vi "HEWH_DSM_CMD.vi"(10 "Command":T1=34 items=["RQST_SOFTWARE_VERSION", "RQST_T2_RESISTANCE", "RQST_T3A_RESISTANCE", "RQST_T3B_RESISTANCE", "RQST_T4_RESISTANCE", "RQST_T5_RESISTANCE", "RQST_IDLB_RESISTANCE", "RQST_MODE_SELECT_RESISTANCE", "RQST_DATA_FROM_MEMORY", "RQST_DATA_FROM_DATA_FLASH", "RQST_SS_FAULT_COUNTS", "RQST_OTHER_FAULT_COUNTS", "CMD_CLEAR_FAULT_COUNTS", "RQST_HYPERTERM_OUTPUT_DATA", "CMD_RESET_FILTER_TIMES", "CMD_WRITE_SETPOINTS", "CMD_TURN_ON_OFF_DLB", "CMD_ENTER_EXIT_FCT_MODE", "CMD_SET_LEDS", "CMD_SET_EEV_DRIVE_LINES", "REQ_READ_KEY_STATUS", "RQST_READ_PERSONALITY", "CMD_ENTER_FACT_MODE", "CMD_RESET", "CMD_RESTORE_EEPROM_DEFAULTS", "CMD_SET_MODEL_NUMBER", "CMD_SET_SERIAL_NUMBER", "RQST_MODEL_NUMBER", "RQST_SERIAL_NUMBER", "CMD_TOGGLE_SERVICE_MODE", "CMD_TOGGLE_UE_SERV", "CMD_TOGGLE_LE_SERV", "CMD_REFRESH_SERVICE_TIMEOUTS", "RQST_DSM_OVERRIDE_STATUS", "RQST_STATUS_QUERY", "RQST_HEM_KWH_DATA", "RQST_SERVICE_ERROR_CODES", "RQST_OVERRIDE_STATUS", "CMD_UPDATE_DSM_LEVEL", "CMD_OVERRIDE_STATUS_CHANGED", "CMD_CLEAR_OVERRIDE_STATUS", "CMD_CLEAR_ENERGY_USAGE_CTRS", "CMD_DSM_OVERRIDES", "CMD_UPDATE_MODE", "CMD_SET_PID_P_DENOMINATOR", "CMD_SET_PID_I_DENOM_UNDER_THR", "CMD_SET_PID_I_DENOM_OVER_THR", "CMD_SET_START_POS_UNDER_THR", "CMD_SET_START_POS_OVER_THR", "CMD_SET_EEV_STOP_POSITION", "CMD_SET_AMBIENT_THRESH_1", "CMD_SET_AMBIENT_THRESH_2", "CMD_SET_AMBIENT_THRESH_3", "CMD_SET_PID_LOW_SH_TARGET", "CMD_SET_PID_MID_SH_TARGET", "RQST_PID_PARAMETERS", "CMD_COMP_OFF", "CMD_TOGGLE_FAN", "CMD_RQST_LED_STATUS", "CMD_UE_2_SECONDS", "CMD_LE_2_SECONDS", "CMD_COMP_ON", "CMD_HP_RUN_6MIN", "RQST_TEMP_RANGE", "RQST_VACATION_RANGE", "RQST_STD_ELEC_RANGE", "RQST_WATER_CAPACITY", "CMD_CANCEL_EEV_POSITION", "CMD_EEV_POSITION", "CMD_SET_CURRENTS", "RQST_SUPPORTED_MODES"]) -> (2 "CMD Array":u8[](array[numeric])=[222, 2] format="%02x")   [LabVIEW 2009]
uses:
  HEWH Command Type.ctl
panel:
  in  "Commands":cluster{"String":string, "CMD Array":u8[]}[](array[cluster])=[{"String"="RQST_SOFTWARE_VERSION", "CMD Array"=[1]}, {"String"="RQST_T2_RESISTANCE", "CMD Array"=[16]}, {"String"="RQST_T3A_RESISTANCE", "CMD Array"=[17]}, {"String"="RQST_T3B_RESISTANCE", "CMD Array"=[18]}, {"String"="RQST_T4_RESISTANCE", "CMD Array"=[19]}, {"String"="RQST_T5_RESISTANCE", "CMD Array"=[20]}, {"String"="RQST_IDLB_RESISTANCE", "CMD Array"=[21]}, {"String"="RQST_MODE_SELECT_RESISTANCE", "CMD Array"=[22]}, {"String"="RQST_DATA_FROM_MEMORY", "CMD Array"=[78]}, {"String"="RQST_DATA_FROM_DATA_FLASH", "CMD Array"=[79]}, {"String"="RQST_SS_FAULT_COUNTS", "CMD Array"=[83]}, {"String"="RQST_OTHER_FAULT_COUNTS", "CMD Array"=[84]}, {"String"="CMD_CLEAR_FAULT_COUNTS", "CMD Array"=[85]}, {"String"="RQST_HYPERTERM_OUTPUT_DATA", "CMD Array"=[86]}, {"String"="CMD_RESET_FILTER_TIMES", "CMD Array"=[144]}, {"String"="CMD_WRITE_SETPOINTS", "CMD Array"=[165]}, {"String"="CMD_TURN_ON_OFF_DLB", "CMD Array"=[176]}, {"String"="CMD_ENTER_EXIT_FCT_MODE", "CMD Array"=[180]}, {"String"="CMD_SET_LEDS", "CMD Array"=[181]}, {"String"="CMD_SET_EEV_DRIVE_LINES", "CMD Array"=[182]}, {"String"="REQ_READ_KEY_STATUS", "CMD Array"=[183]}, {"String"="RQST_READ_PERSONALITY", "CMD Array"=[188]}, {"String"="CMD_ENTER_FACT_MODE", "CMD Array"=[192]}, {"String"="CMD_RESET", "CMD Array"=[193]}, {"String"="CMD_RESTORE_EEPROM_DEFAULTS", "CMD Array"=[194]}, {"String"="CMD_SET_MODEL_NUMBER", "CMD Array"=[195]}, {"String"="CMD_SET_SERIAL_NUMBER", "CMD Array"=[196]}, {"String"="RQST_MODEL_NUMBER", "CMD Array"=[197]}, {"String"="RQST_SERIAL_NUMBER", "CMD Array"=[198]}, {"String"="CMD_TOGGLE_SERVICE_MODE", "CMD Array"=[200]}, {"String"="CMD_TOGGLE_UE_SERV", "CMD Array"=[201]}, {"String"="CMD_TOGGLE_LE_SERV", "CMD Array"=[202]}, {"String"="CMD_REFRESH_SERVICE_TIMEOUTS", "CMD Array"=[203]}, {"String"="RQST_DSM_OVERRIDE_STATUS", "CMD Array"=[222, 2]}, {"String"="RQST_STATUS_QUERY", "CMD Array"=[222, 16]}, {"String"="RQST_HEM_KWH_DATA", "CMD Array"=[222, 18]}, {"String"="RQST_SERVICE_ERROR_CODES", "CMD Array"=[222, 20]}, {"String"="RQST_OVERRIDE_STATUS", "CMD Array"=[222, 23]}, {"String"="CMD_UPDATE_DSM_LEVEL", "CMD Array"=[223, 0]}, {"String"="CMD_OVERRIDE_STATUS_CHANGED", "CMD Array"=[223, 2]}, {"String"="CMD_CLEAR_OVERRIDE_STATUS", "CMD Array"=[223, 3]}, {"String"="CMD_CLEAR_ENERGY_USAGE_CTRS", "CMD Array"=[223, 7]}, {"String"="CMD_DSM_OVERRIDES", "CMD Array"=[223, 19]}, {"String"="CMD_UPDATE_MODE", "CMD Array"=[223, 20]}, {"String"="CMD_SET_PID_P_DENOMINATOR", "CMD Array"=[0]}, {"String"="CMD_SET_PID_I_DENOM_UNDER_THR", "CMD Array"=[0]}, {"String"="CMD_SET_PID_I_DENOM_OVER_THR", "CMD Array"=[0]}, {"String"="CMD_SET_START_POS_UNDER_THR", "CMD Array"=[0]}, {"String"="CMD_SET_START_POS_OVER_THR", "CMD Array"=[0]}, {"String"="CMD_SET_EEV_STOP_POSITION", "CMD Array"=[0]}, {"String"="CMD_SET_AMBIENT_THRESH_1", "CMD Array"=[0]}, {"String"="CMD_SET_AMBIENT_THRESH_2", "CMD Array"=[0]}, {"String"="CMD_SET_AMBIENT_THRESH_3", "CMD Array"=[0]}, {"String"="CMD_SET_PID_LOW_SH_TARGET", "CMD Array"=[0]}, {"String"="CMD_SET_PID_MID_SH_TARGET", "CMD Array"=[0]}, {"String"="RQST_PID_PARAMETERS", "CMD Array"=[0]}, {"String"="CMD_COMP_OFF", "CMD Array"=[240]}, {"String"="CMD_TOGGLE_FAN", "CMD Array"=[241]}, {"String"="CMD_RQST_LED_STATUS", "CMD Array"=[242]}, {"String"="CMD_UE_2_SECONDS", "CMD Array"=[243]}, {"String"="CMD_LE_2_SECONDS", "CMD Array"=[244]}, {"String"="CMD_COMP_ON", "CMD Array"=[245]}, {"String"="CMD_HP_RUN_6MIN", "CMD Array"=[246]}, {"String"="RQST_TEMP_RANGE", "CMD Array"=[247]}, {"String"="RQST_VACATION_RANGE", "CMD Array"=[248]}, {"String"="RQST_STD_ELEC_RANGE", "CMD Array"=[249]}, {"String"="RQST_WATER_CAPACITY", "CMD Array"=[250]}, {"String"="CMD_CANCEL_EEV_POSITION", "CMD Array"=[251]}, {"String"="CMD_EEV_POSITION", "CMD Array"=[252]}, {"String"="CMD_SET_CURRENTS", "CMD Array"=[253]}, {"String"="RQST_SUPPORTED_MODES", "CMD Array"=[254]}] {"CMD Array" format="%.0x"}
  out "Data Array":string[][](array[string])=[["CMD_WRITE_SETPOINTS", "0x60", "0xA5", "N/A", "Any"], ["RQST_NON_CRIT_VERSION", "0x60", "0x01", "N/A", "Any"], ["RQST_CRIT_VERSION", "0x60", "0x02", "N/A", "Any"], ["RQST_EEPROM_VERSION", "0x60", "0x03", "N/A", "Any"], ["RQST_T2_RESISTANCE", "0x60", "0x10", "N/A", "Any"], ["RQST_T3A_RESISTANCE", "0x60", "0x11", "N/A", "Any"], ["RQST_T3B_RESISTANCE", "0x60", "0x12", "N/A", "Any"], ["RQST_T4_RESISTANCE", "0x60", "0x13", "N/A", "Any"], ["RQST_T5_RESISTANCE", "0x60", "0x14", "N/A", "Any"], ["RQST_IDLB_RESISTANCE", "0x60", "0x15", "N/A", "Any"], ["RQST_MODE_SELECT_RESISTANCE", "0x60", "0x16", "N/A", "Any"], ["RQST_STATUS INFO", "0x60", "0x50", "N/A", "Any"], ["RQST_SS_FAULT_COUNTS", "0x60", "0x53", "N/A", "Any"], ["RQST_OTHER_FAULT_COUNTS", "0x60", "0x54", "N/A", "Any"], ["CMD_CLEAR_FAULT_COUNTS", "0x60", "0x55", "N/A", "Any"], ["RQST_HYPERTERM_OUTPUT_DATA", "0x60", "0x56", "N/A", "Any"], ["RQST_READ_PERSONALITY", "0x60", "0xBC", "N/A", "Any"], ["RQST_DSM_OVERRIDE_STATUS", "0x60", "0xDE", "0x02", "Any"], ["RQST_STATUS_QUERY", "0x60", "0xDE", "0x10", "Any"], ["RQST_HEM_KWH_DATA", "0x60", "0xDE", "0x12", "Any"], ["RQST_SERVICE_ERROR_CODES", "0x60", "0xDE", "0x14", "Any"], ["RQST_OVERRIDE_STATUS", "0x60", "0xDE", "0x17", "Any"], ["CMD_CLEAR_OVERRIDE_STATUS", "0x60", "0xDF", "0x03", "0x40"], ["CMD_CLEAR_ENERGY_USAGE_CTRS", "0x60", "0xDF", "0x07", "0x40"], ["CMD_COMP_OFF", "0x60", "0xF0", "N/A", "Any"], ["CMD_UE_2_SECONDS", "0x60", "0xF3", "N/A", "Any"], ["CMD_LE_2_SECONDS", "0x60", "0xF4", "N/A", "Any"], ["CMD_COMP_ON", "0x60", "0xF5", "N/A", "Any"], ["CMD_HP_RUN_6MIN", "0x60", "0xF6", "N/A", "Any"], ["RQST_TEMP_RANGE", "0x60", "0xF7", "N/A", "Any"], ["RQST_VACATION_RANGE", "0x60", "0xF8", "N/A", "Any"], ["RQST_STD_ELEC_RANGE", "0x60", "0xF9", "N/A", "Any"], ["RQST_WATER_CAPACITY", "0x60", "0xFA", "N/A", "Any"], ["CMD_CANCEL_EEV_POSITION", "0x60", "0xFB", "N/A", "Any"], ["RQST_SUPPORTED_MODES", "0x60", "0xFE", "N/A", "Any"], ["CMD_CONTROL_FAN1", "0x60", "0xF1", "N/A", "Any"], ["CMD_EEV_POSITION", "0x60", "0xFC", "N/A", "Any"], ["CMD_SET_EEV_START_POSITION", "0x60", "E5", "N/A", "Any"], ["CMD_SET_EEV_STOP_POSITION", "0x60", "EA", "N/A", "Any"], ["CMD_UPDATE_DSM_LEVEL", "0x60", "0xDF", "0x00", "0x40"], ["CMD_SET_PID_I_DENOMINATOR", "0x60", "E3", "N/A", "Any"], ["CMD_SET_PID_I_NUMERATOR", "0x60", "E2", "N/A", "Any"], ["RQST_DATA_FROM_MEMORY", "0x60", "0x4E", "N/A", "Any"], ["CMD_OVERRIDE_STATUS_CHANGED", "0x40", "0xDF", "0x02", "0x60"], ["CMD_SET_PID_P_DENOMINATOR", "0x60", "E1", "N/A", "Any"], ["CMD_SET_PID_P_NUMERATOR", "0x60", "E0", "N/A", "Any"], ["CMD_SET_PID_RUN_SH_TARGET", "0x60", "E9", "N/A", "Any"], ["CMD_SET_PID_START_DWELL_TIME", "0x60", "E6", "N/A", "Any"], ["CMD_SET_PID_TRANSITION_TIME", "0x60", "E8", "N/A", "Any"], ["CMD_SET_PID_TRANS_SH_TARGET", "0x60", "E7", "N/A", "Any"], ["CMD_SET_PID_UPDATE_RATE", "0x60", "E4", "N/A", "Any"], ["RQST_DATA_FROM_DATA_FLASH", "0x60", "0x4F", "N/A", "Any"], ["CMD_DSM_OVERRIDES", "0x60", "0xDF", "0x13", "Any"], ["CMD_UPDATE_MODE", "0x60", "0xDF", "0x14", "Any"], ["CMD_UPDATE_SPECIAL_OPERATION", "0x60", "0xDF", "0x15", "Any"], ["CMD_SET_CURRENTS", "0x60", "0xFD", "N/A", "Any"], ["CMD_RESET_FILTER_TIMES", "0x60", "0x90", "N/A", "Any"], ["CMD_TURN_ON_DLB", "0x60", "B0", "N/A", "Any"], ["RQST_PID_PARAMETERS", "0x60", "EF", "N/A", "Any"], ["CMD_CHECK_CRC", "0x60", "0xA6", "N/A", "Any"], ["CMD_ENTER_FACT_MODE", "0x60", "0xC0", "N/A", "Any"], ["CMD_RESET", "0x60", "0xC1", "N/A", "Any"], ["CMD_RESTORE_EEPROM_DEFAULTS", "0x60", "0xC2", "N/A", "Any"]]
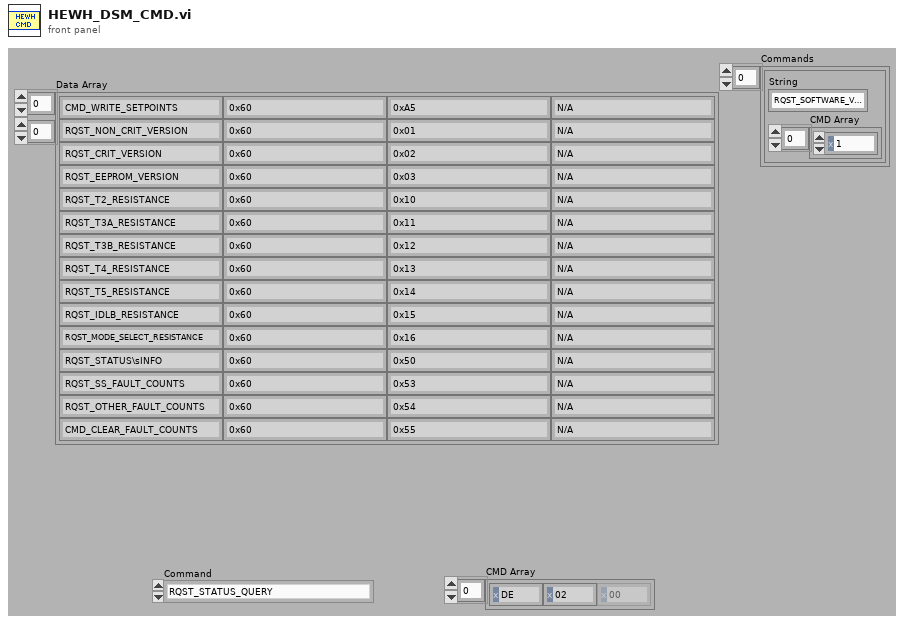
[diagram p1: front panel]
types:
  T1 = typedef "HEWH Command Type.ctl" = u8
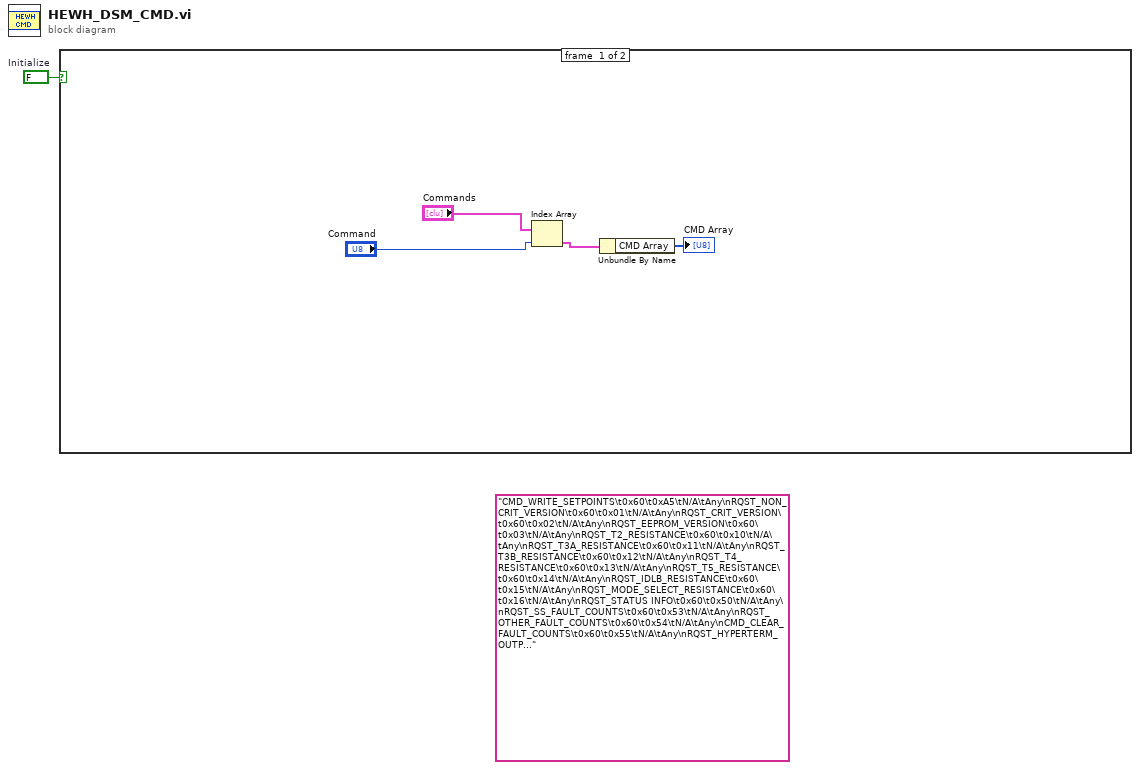
[diagram p0: block diagram]
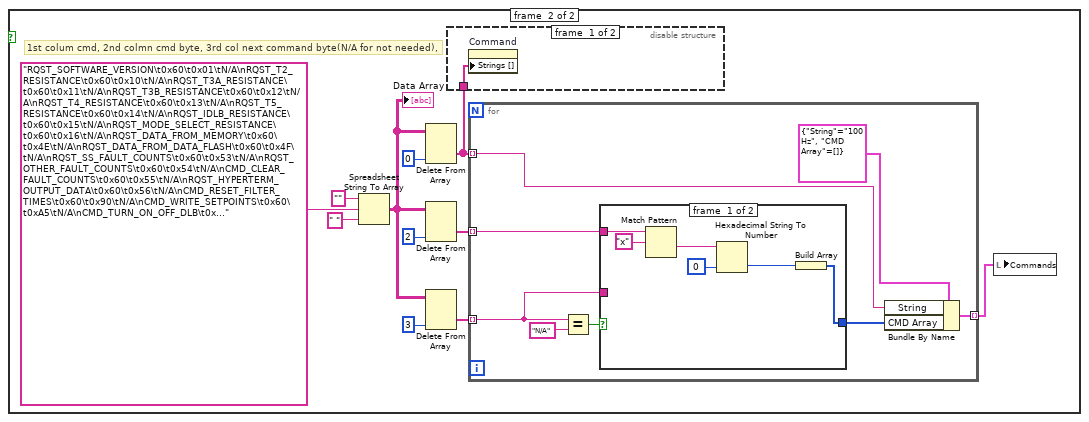
[diagram p2: hidden frame]
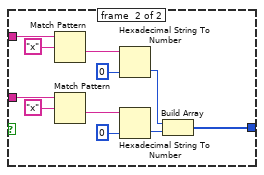
[diagram p4: hidden frame]
diagram:
  (unwired) "CMD_WRITE_SETPOINTS\t0x60\t0xA5\tN/A\tAny\nRQST_NON_CRIT_VERSION\t0x60\t0x01\tN/A\tAny\nRQST_CRIT_VERSION\t0x60\t0x02\tN/A\tAny\nRQST_EEPROM_VERSION\t0x60\t0x03\tN/A\tAny\nRQST_T2_RESISTANCE\t0x60\t0x10\tN/A\tAny\nRQST_T3A_RESISTANCE\t0x60\t0x11\tN/A\tAny\nRQST_T3B_RESISTANCE\t0x60\t0x12\tN/A\tAny\nRQST_T4_RESISTANCE\t0x60\t0x13\tN/A\tAny\nRQST_T5_RESISTANCE\t0x60\t0x14\tN/A\tAny\nRQST_IDLB_RESISTANCE\t0x60\t0x15\tN/A\tAny\nRQST_MODE_SELECT_RESISTANCE\t0x60\t0x16\tN/A\tAny\nRQST_STATUS INFO\t0x60\t0x50\tN/A\tAny\nRQST_SS_FAULT_COUNTS\t0x60\t0x53\tN/A\tAny\nRQST_OTHER_FAULT_COUNTS\t0x60\t0x54\tN/A\tAny\nCMD_CLEAR_FAULT_COUNTS\t0x60\t0x55\tN/A\tAny\nRQST_HYPERTERM_OUTPUT_DATA\t0x60\t0x56\tN/A\tAny\nRQST_READ_PERSONALITY\t0x60\t0xBC\tN/A\tAny\nRQST_DSM_OVERRIDE_STATUS\t0x60\t0xDE\t0x02\tAny\nRQST_STATUS_QUERY\t0x60\t0xDE\t0x10\tAny\nRQST_HEM_KWH_DATA\t0x60\t0xDE\t0x12\tAny\nRQST_SERVICE_ERROR_CODES\t0x60\t0xDE\t0x14\tAny\nRQST_OVERRIDE_STATUS\t0x60\t0xDE\t0x17\tAny\nCMD_CLEAR_OVERRIDE_STATUS\t0x60\t0xDF\t0x03\t0x40\nCMD_CLEAR_ENERGY_USAGE_CTRS\t0x60\t0xDF\t0x07\t0x40\nCMD_COMP_OFF\t0x60\t0xF0\tN/A\tAny\nCMD_UE_2_SECONDS\t0x60\t0xF3\tN/A\tAny\nCMD_LE_2_SECONDS\t0x60\t0xF4\tN/A\tAny\nCMD_COMP_ON\t0x60\t0xF5\tN/A\tAny\nCMD_HP_RUN_6MIN\t0x60\t0xF6\tN/A\tAny\nRQST_TEMP_RANGE\t0x60\t0xF7\tN/A\tAny\nRQST_VACATION_RANGE\t0x60\t0xF8\tN/A\tAny\nRQST_STD_ELEC_RANGE\t0x60\t0xF9\tN/A\tAny\nRQST_WATER_CAPACITY\t0x60\t0xFA\tN/A\tAny\nCMD_CANCEL_EEV_POSITION\t0x60\t0xFB\tN/A\tAny\nRQST_SUPPORTED_MODES\t0x60\t0xFE\tN/A\tAny\nCMD_CONTROL_FAN1\t0x60\t0xF1\tN/A\tAny\nCMD_EEV_POSITION\t0x60\t0xFC\tN/A\tAny\nCMD_SET_EEV_START_POSITION\t0x60\tE5\tN/A\tAny\nCMD_SET_EEV_STOP_POSITION\t0x60\tEA\tN/A\tAny\nCMD_UPDATE_DSM_LEVEL\t0x60\t0xDF\t0x00\t0x40\nCMD_SET_PID_I_DENOMINATOR\t0x60\tE3\tN/A\tAny\nCMD_SET_PID_I_NUMERATOR\t0x60\tE2\tN/A\tAny\nRQST_DATA_FROM_MEMORY\t0x60\t0x4E\tN/A\tAny\nCMD_OVERRIDE_STATUS_CHANGED\t0x40\t0xDF\t0x02\t0x60\nCMD_SET_PID_P_DENOMINATOR\t0x60\tE1\tN/A\tAny\nCMD_SET_PID_P_NUMERATOR\t0x60\tE0\tN/A\tAny\nCMD_SET_PID_RUN_SH_TARGET\t0x60\tE9\tN/A\tAny\nCMD_SET_PID_START_DWELL_TIME\t0x60\tE6\tN/A\tAny\nCMD_SET_PID_TRANSITION_TIME\t0x60\tE8\tN/A\tAny\nCMD_SET_PID_TRANS_SH_TARGET\t0x60\tE7\tN/A\tAny\nCMD_SET_PID_UPDATE_RATE\t0x60\tE4\tN/A\tAny\nRQST_DATA_FROM_DATA_FLASH\t0x60\t0x4F\tN/A\tAny\nCMD_DSM_OVERRIDES\t0x60\t0xDF\t0x13\tAny\nCMD_UPDATE_MODE\t0x60\t0xDF\t0x14\tAny\nCMD_UPDATE_SPECIAL_OPERATION\t0x60\t0xDF\t0x15\tAny\nCMD_SET_CURRENTS\t0x60\t0xFD\tN/A\tAny\nCMD_RESET_FILTER_TIMES\t0x60\t0x90\tN/A\tAny\nCMD_TURN_ON_DLB\t0x60\tB0\tN/A\tAny\nRQST_PID_PARAMETERS\t0x60\tEF\tN/A\tAny\nCMD_CHECK_CRC\t0x60\t0xA6\tN/A\tAny\nCMD_ENTER_FACT_MODE\t0x60\t0xC0\tN/A\tAny\nCMD_RESET\t0x60\t0xC1\tN/A\tAny\nCMD_RESTORE_EEPROM_DEFAULTS\t0x60\t0xC2\tN/A\tAny\n"
  w1 = FALSE  # Initialize
  n1 = case shown="True" w1 {
    frame #0 {
      n2 = Index Array(array="Commands", index="Command") -> (element=w3:cluster{"String":string, "CMD Array":u8[]})
      n3 = Unbundle By Name(w3) -> ("CMD Array"=→"CMD Array":u8[])
    }
    frame #1 {
      # "1st colum cmd, 2nd colmn cmd byte, 3rd col next command byte(N/A for not needed),"
      n4 = Spreadsheet String To Array(format string="", spreadsheet string="RQST_SOFTWARE_VERSION\t0x60\t0x01\tN/A\nRQST_T2_RESISTANCE\t0x60\t0x10\tN/A\nRQST_T3A_RESISTANCE\t0x60\t0x11\tN/A\nRQST_T3B_RESISTANCE\t0x60\t0x12\tN/A\nRQST_T4_RESISTANCE\t0x60\t0x13\tN/A\nRQST_T5_RESISTANCE\t0x60\t0x14\tN/A\nRQST_IDLB_RESISTANCE\t0x60\t0x15\tN/A\nRQST_MODE_SELECT_RESISTANCE\t0x60\t0x16\tN/A\nRQST_DATA_FROM_MEMORY\t0x60\t0x4E\tN/A\nRQST_DATA_FROM_DATA_FLASH\t0x60\t0x4F\tN/A\nRQST_SS_FAULT_COUNTS\t0x60\t0x53\tN/A\nRQST_OTHER_FAULT_COUNTS\t0x60\t0x54\tN/A\nCMD_CLEAR_FAULT_COUNTS\t0x60\t0x55\tN/A\nRQST_HYPERTERM_OUTPUT_DATA\t0x60\t0x56\tN/A\nCMD_RESET_FILTER_TIMES\t0x60\t0x90\tN/A\nCMD_WRITE_SETPOINTS\t0x60\t0xA5\tN/A\nCMD_TURN_ON_OFF_DLB\t0x60\t0xB0\tN/A\nCMD_ENTER_EXIT_FCT_MODE\t0x60\t0xB4\tN/A\nCMD_SET_LEDS\t0x60\t0xB5\tN/A\nCMD_SET_EEV_DRIVE_LINES\t0x60\t0xB6\tN/A\nREQ_READ_KEY_STATUS\t0x60\t0xB7\tN/A\nRQST_READ_PERSONALITY\t0x60\t0xBC\tN/A\nCMD_ENTER_FACT_MODE\t0x60\t0xC0\tN/A\nCMD_RESET\t0x60\t0xC1\tN/A\nCMD_RESTORE_EEPROM_DEFAULTS\t0x60\t0xC2\tN/A\nCMD_SET_MODEL_NUMBER\t0x60\t0xC3\tN/A\nCMD_SET_SERIAL_NUMBER\t0x60\t0xC4\tN/A\nRQST_MODEL_NUMBER\t0x60\t0xC5\tN/A\nRQST_SERIAL_NUMBER\t0x60\t0xC6\tN/A\nCMD_TOGGLE_SERVICE_MODE\t0x60\t0xC8\tN/A\nCMD_TOGGLE_UE_SERV\t0x60\t0xC9\tN/A\nCMD_TOGGLE_LE_SERV\t0x60\t0xCA\tN/A\nCMD_REFRESH_SERVICE_TIMEOUTS\t0x60\t0xCB\tN/A\nRQST_DSM_OVERRIDE_STATUS\t0x60\t0xDE\t0x02\nRQST_STATUS_QUERY\t0x60\t0xDE\t0x10\nRQST_HEM_KWH_DATA\t0x60\t0xDE\t0x12\nRQST_SERVICE_ERROR_CODES\t0x60\t0xDE\t0x14\nRQST_OVERRIDE_STATUS\t0x60\t0xDE\t0x17\nCMD_UPDATE_DSM_LEVEL\t0x60\t0xDF\t0x00\nCMD_OVERRIDE_STATUS_CHANGED\t0x40\t0xDF\t0x02\nCMD_CLEAR_OVERRIDE_STATUS\t0x60\t0xDF\t0x03\nCMD_CLEAR_ENERGY_USAGE_CTRS\t0x60\t0xDF\t0x07\nCMD_DSM_OVERRIDES\t0x60\t0xDF\t0x13\nCMD_UPDATE_MODE\t0x60\t0xDF\t0x14\nCMD_SET_PID_P_DENOMINATOR\t0x60\tE0\tN/A\nCMD_SET_PID_I_DENOM_UNDER_THR\t0x60\tE1\tN/A\nCMD_SET_PID_I_DENOM_OVER_THR\t0x60\tE2\tN/A\nCMD_SET_START_POS_UNDER_THR\t0x60\tE3\tN/A\nCMD_SET_START_POS_OVER_THR\t0x60\tE4\tN/A\nCMD_SET_EEV_STOP_POSITION\t0x60\tE5\tN/A\nCMD_SET_AMBIENT_THRESH_1\t0x60\tE6\tN/A\nCMD_SET_AMBIENT_THRESH_2\t0x60\tE7\tN/A\nCMD_SET_AMBIENT_THRESH_3\t0x60\tE8\tN/A\nCMD_SET_PID_LOW_SH_TARGET\t0x60\tE9\tN/A\nCMD_SET_PID_MID_SH_TARGET\t0x60\tEA\tN/A\nRQST_PID_PARAMETERS\t0x60\tEF\tN/A\nCMD_COMP_OFF\t0x60\t0xF0\tN/A\nCMD_TOGGLE_FAN\t0x60\t0xF1\tN/A\nCMD_RQST_LED_STATUS\t0x60\t0xF2\tN/A\nCMD_UE_2_SECONDS\t0x60\t0xF3\tN/A\nCMD_LE_2_SECONDS\t0x60\t0xF4\tN/A\nCMD_COMP_ON\t0x60\t0xF5\tN/A\nCMD_HP_RUN_6MIN\t0x60\t0xF6\tN/A\nRQST_TEMP_RANGE\t0x60\t0xF7\tN/A\nRQST_VACATION_RANGE\t0x60\t0xF8\tN/A\nRQST_STD_ELEC_RANGE\t0x60\t0xF9\tN/A\nRQST_WATER_CAPACITY\t0x60\t0xFA\tN/A\nCMD_CANCEL_EEV_POSITION\t0x60\t0xFB\tN/A\nCMD_EEV_POSITION\t0x60\t0xFC\tN/A\nCMD_SET_CURRENTS\t0x60\t0xFD\tN/A\nRQST_SUPPORTED_MODES\t0x60\t0xFE\tN/A\n", array type (2D Dbl)=" " ("delimiter (Tab)")) -> (array=w9:string[][])  [unwired: 1 in]
      "Data Array" <- w9
      n5 = Delete From Array(array=w9, index (col)=0 ("disabled index (col)")) -> (deleted portion=w13:string[])  [unwired: 2 in, 1 out]
      n6 = Delete From Array(array=w9, index (col)=2 ("disabled index (col)")) -> (deleted portion=w11:string[])  [unwired: 2 in, 1 out]
      n7 = Delete From Array(array=w9, index (col)=3 ("disabled index (col)")) -> (deleted portion=w8:string[])  [unwired: 2 in, 1 out]
      n8 = disable-structure shown="Enabled" {
        disable-tunnel: w13 -> [w17 _]
        frame #0 {
          n9 = property on="Command" class="Ring (strict)"("Strings []"=w17) -> ()  [unwired: 2 in, 2 out]
        }
        frame #1 {
          # "Enable to update typedef."
        }
      }
      n10 = for {
        tunnel: w13 -> [w24] mode=indexing
        tunnel: w11 -> [w23] mode=indexing
        tunnel: [w22] -> w7 mode=indexing
        tunnel: w8 -> [w18] mode=indexing
        n11 = Equal?(x=w18, y="N/A") -> (x = y?=w19:bool)
        n12 = case shown="False" w19 {
          tunnel: w23 -> [w31 w42]
          tunnel: [w26 w38] -> w21
          tunnel: w18 -> [_ w36]
          frame #0 {
            n13 = Match Pattern(string=w31, regular expression="x") -> (after substring=w29:string)  [unwired: 1 in, 3 out]
            n14 = Hexadecimal String To Number(string=w29, default (0uL)=u8 0 ("default (0 U32)")) -> (number=w27:u8)  [unwired: 1 in, 1 out]
            n15 = Build Array(w27) -> (w26:u8[])
          }
          frame #1 {
            n16 = Match Pattern(string=w42, regular expression="x") -> (after substring=w40:string)  [unwired: 1 in, 3 out]
            n17 = Match Pattern(string=w36, regular expression="x") -> (after substring=w33:string)  [unwired: 1 in, 3 out]
            n18 = Hexadecimal String To Number(string=w40, default (0uL)=u8 0 ("default (0 U32)")) -> (number=w39:u8)  [unwired: 1 in, 1 out]
            n19 = Hexadecimal String To Number(string=w33, default (0uL)=u8 0 ("default (0 U32)")) -> (number=w32:u8)  [unwired: 1 in, 1 out]
            n20 = Build Array(w39, w32) -> (w38:u8[])
          }
        }
        n21 = Bundle By Name(cluster=cluster{"String":string, "CMD Array":u8[]} {"String"="100 Hz", "CMD Array"=[]}, "String"=w24, "CMD Array"=w21) -> (w22:cluster{"String":string, "CMD Array":u8[]})
      }
      n22 = local write "Commands"(w7) -> ()
    }
  }
